vi "CPU_MEM_Color.vi"(5 "read all":bool, 7 "oper":enum16{"init", "read", "write"}(ring), 10 "value in":u8 format="%02x", 11 "address":u16 format="%04x") -> (2 "value out":u8 format="%02x", 3 "mem":u8[](array[numeric])=[27, 8, 14, 6, 20] format="%02x")   [LabVIEW 2018]
panel:
  in  "init size":u16=1023 format="%.0x"
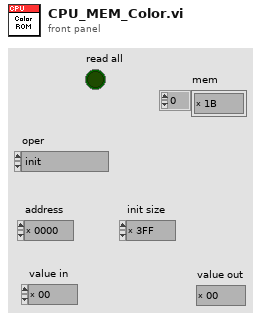
[diagram p1: front panel]
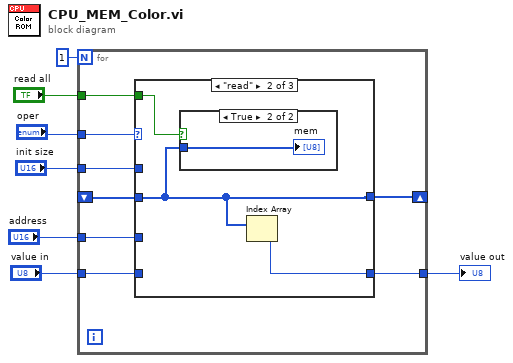
[diagram p0: block diagram]
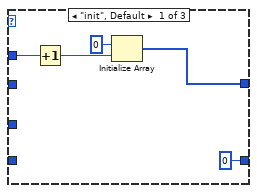
[diagram p2: hidden frame]
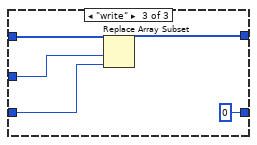
[diagram p4: hidden frame]
diagram:
  n1 = for {
    N: 1 -> [_]
    shift-right: [w13] -> _
    shift-left: _ -> [w12]
    tunnel: "oper" -> [w15]
    tunnel: "init size" -> [w14]
    tunnel: [w11] -> w4
    tunnel: "address" -> [w10]
    tunnel: "value in" -> [w9]
    tunnel: "read all" -> [w8]
    n2 = case shown="\"read\"" w15 {
      tunnel: w14 -> [w20 _ _]
      tunnel: [w18 w21 w26] -> w13
      tunnel: w12 -> [_ w21 w29]
      tunnel: [u8 0 ("element") w23 u8 0 ("element")] -> w11
      tunnel: w10 -> [_ _ w28]
      tunnel: w9 -> [_ _ w27]
      tunnel: w8 -> [_ w22 _]
      frame "init", Default {
        n3 = Increment(x=w20) -> (x+1=w16:u16)
        n4 = Initialize Array(u8 0 ("element"), w16) -> (w18:u8[])
      }
      frame "read" {
        n5 = case shown="True" w22 {
          tunnel: w21 -> [_ w24]
          frame False {
          }
          frame True {
            "mem" <- w24
          }
        }
        n6 = Index Array(array=w21) -> (element=w23:u8)  [unwired: 1 in]
      }
      frame "write" {
        n7 = Replace Array Subset(array=w29, new element=w27, index=w28) -> (w26:u8[])
      }
    }
  }
  "value out" <- w4
